vi "Unpack serial array.vi"(11 "Array":string[](array[string])) -> (0 "write data?":bool, 1 "Cluster 2":T1, 2 "Array[10]":string, 3 "Waveform Out":waveform(i32), 4 "Cluster":T2, 5 "current time":timestamp, 7 "Numeric":i32)   [LabVIEW 2016]
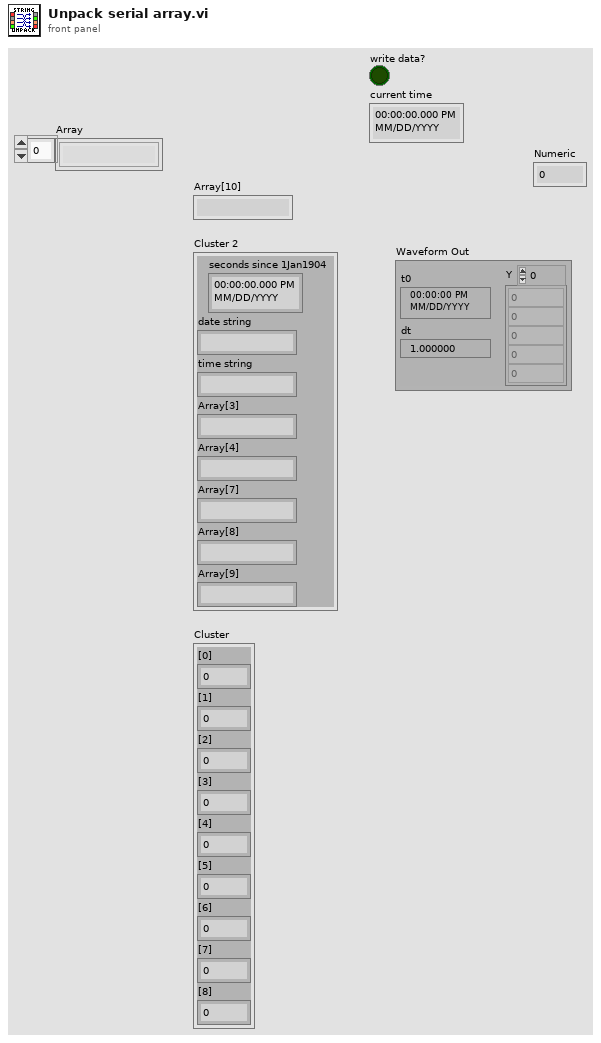
[diagram p1: front panel]
types:
  T1 = cluster{"seconds since 1Jan1904":timestamp, "date string":string, "time string":string, "Array[3]":string, "Array[4]":string, "Array[7]":string, "Array[8]":string, "Array[9]":string}
  T2 = cluster{"[0]":dbl, "[1]":dbl, "[2]":dbl, "[3]":dbl, "[4]":dbl, "[5]":dbl, "[6]":dbl, "[7]":dbl, "[8]":dbl}
  T3 = cluster{"Array[0]":string, "Array[1]":string, "Array[2]":string, "Array[3]":string, "Array[4]":string, "Array[5]":string, "Array[6]":string, "Array[7]":string, "Array[8]":string, "Array[9]":string, "Array[10]":string}
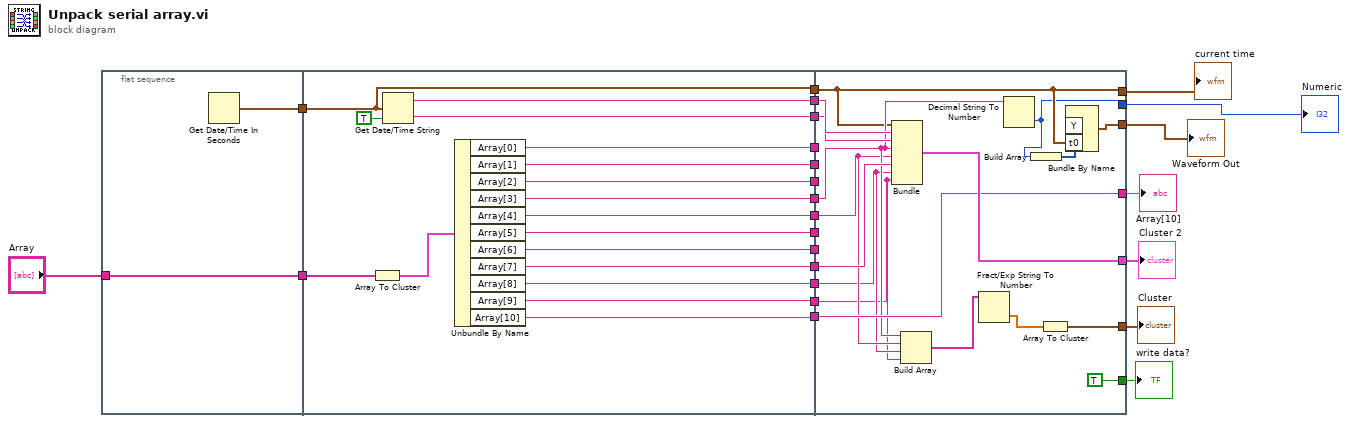
[diagram p0: block diagram]
diagram:
  n1 = flat-sequence {
    tunnel: [w26] -> w24
    tunnel: "Array" -> [w25]
    tunnel: [w25] -> w23
    tunnel: w24 -> [w41]
    tunnel: w23 -> [w42]
    tunnel: [w41] -> w22
    tunnel: [w40] -> w21
    tunnel: [w39] -> w20
    tunnel: [w38] -> w19
    tunnel: [w37] -> w18
    tunnel: [w36] -> w17
    tunnel: [w35] -> w16
    tunnel: [w34] -> w15
    tunnel: [w33] -> w14
    tunnel: [w32] -> w13
    tunnel: [w31] -> w12
    tunnel: [w30] -> w11
    tunnel: [w29] -> w10
    tunnel: [w28] -> w9
    tunnel: [w60] -> w8
    tunnel: w22 -> [w46]
    tunnel: w21 -> [w59]
    tunnel: w20 -> [w58]
    tunnel: w19 -> [_]
    tunnel: w18 -> [_]
    tunnel: w17 -> [_]
    tunnel: w16 -> [w54]
    tunnel: w15 -> [w53]
    tunnel: w14 -> [_]
    tunnel: w13 -> [_]
    tunnel: w12 -> [w57]
    tunnel: w11 -> [w52]
    tunnel: w10 -> [w51]
    tunnel: w9 -> [w55]
    tunnel: [w56] -> w6
    tunnel: [w45] -> w2
    tunnel: [w55] -> w7
    tunnel: [TRUE] -> w4
    tunnel: [w46] -> w3
    tunnel: [w44] -> w1
    frame #0 {
      n2 = Get Date/Time In Seconds() -> (seconds since 1Jan1904=w26:timestamp)
    }
    frame #1 {
      n3 = Array To Cluster(array=w42) -> (cluster=w27:T3)
      n4 = Get Date/Time String(seconds (now)=w41, want seconds? (F)=TRUE) -> (date string=w40:string, time string=w39:string)  [unwired: 1 in]
      n5 = Unbundle By Name(w27) -> ("Array[0]"=w38:string, "Array[1]"=w37:string, "Array[2]"=w36:string, "Array[3]"=w35:string, "Array[4]"=w34:string, "Array[5]"=w33:string, "Array[6]"=w32:string, "Array[7]"=w31:string, "Array[8]"=w30:string, "Array[9]"=w29:string, "Array[10]"=w28:string)
    }
    frame #2 {
      n6 = Bundle("seconds since 1Jan1904"=w46, "date string"=w59, "time string"=w58, "Array[3]"=w54, "Array[4]"=w53, "Array[7]"=w57, "Array[8]"=w52, "Array[9]"=w51) -> (w56:T1)  [unwired: 1 in]
      n7 = Build Array(w54, w53, w52, w51) -> (w50:string[])
      n8 = Fract/Exp String To Number(string=w50) -> (number=w49:dbl[])  [unwired: 3 in, 1 out]
      n9 = Decimal String To Number(string=w54) -> (number=w44:i32)  [unwired: 2 in, 1 out]
      n10 = Build Array(w44) -> (w47:i32[])
      n11 = Array To Cluster(array=w49) -> (cluster=w60:T2)
      n12 = Bundle By Name("Y"=w47, "t0"=w46) -> (w45:waveform(i32))  [unwired: 1 in]
    }
  }
  "Cluster" <- w8
  "Array[10]" <- w7
  "Cluster 2" <- w6
  "write data?" <- w4
  "current time" <- w3
  "Waveform Out" <- w2
  "Numeric" <- w1
